vi "Create Frame Pattern Script.vi"(8 "error in (no error)":errorcluster, 10 "SPI_FRM_Config":T1 {"Addr" format="%x"; "Data" format="%x"}, 11 "SPI_Frame_Root in":refnum<class "SPI_Frame_Root.lvclass">) -> (0 "error out":errorcluster, 3 "SPI_Frame_Root out":refnum<class "SPI_Frame_Root.lvclass">)   [LabVIEW 2018, in "SPI_Frame_Root.lvclass"]
uses:
  SPI_Frame_Root.lvclass
  Config Read SPI/SPI_FRM_Config.ctl
  Classes/Config_Read/RW_Option.ctl
  Config Read SPI/SPI_Mode.ctl
  Classes/Config_Read/Config_Read_BML.lvclass
  Config Read SPI/Config_Read_SPI.lvclass
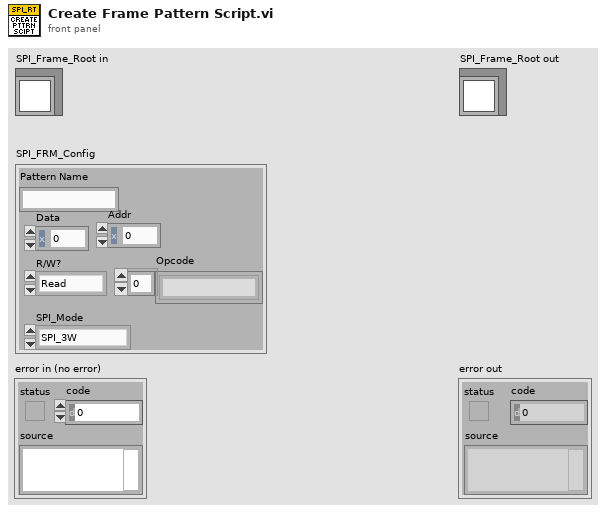
[diagram p1: front panel]
types:
  T1 = typedef "Config_Read_SPI.lvclass/SPI_FRM_Config.ctl" = cluster{"Pattern Name":string, "Data":u16, "Addr":u16, "R/W?":T2, "Opcode":string[], "SPI_Mode":T3}
  T2 = typedef "Config_Read_BML.lvclass/RW_Option.ctl" = enum16{"Read", "Write", "R/W"}
  T3 = typedef "Config_Read_SPI.lvclass/SPI_Mode.ctl" = enum16{"SPI_3W", "SPI_4W"}
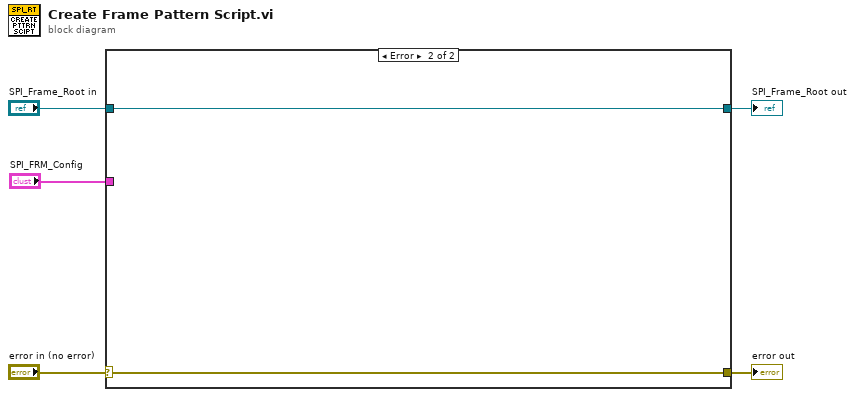
[diagram p0: block diagram]
diagram:
  n1 = case shown="Error" "error in (no error)" {
    selector: "error in (no error)" -> [w6 w9]
    tunnel: [w6 w9] -> w4
    tunnel: [w7 w8] -> w2
    tunnel: "SPI_Frame_Root in" -> [w7 w8]
    tunnel: "SPI_FRM_Config" -> [_ _]
    frame No Error {
      # "Wire the error cluster across even in the \"No Error\"\ncase so that warnings get propagated."
    }
    frame Error {
    }
  }
  "error out" <- w4
  "SPI_Frame_Root out" <- w2
